vi "Get Pole Orientations.vi"(11 "Pole":bool[](array[boolean])) -> (1 "Pole Swap Options Negative":T1, 3 "Pole Swap Options Positive":T1)   [LabVIEW 2018]
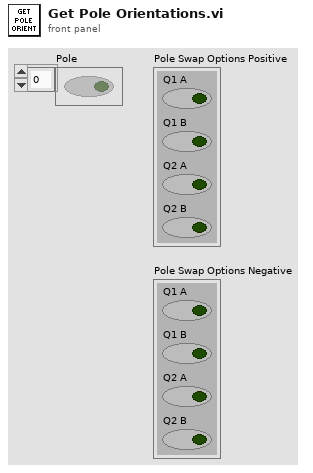
[diagram p1: front panel]
types:
  T1 = cluster{"Q1 A":bool, "Q1 B":bool, "Q2 A":bool, "Q2 B":bool}
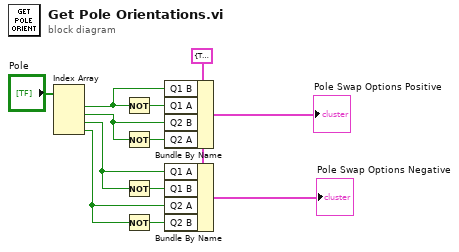
[diagram p0: block diagram]
diagram:
  w12 = T1 {"Q1 A"=TRUE, "Q1 B"=FALSE, "Q2 A"=TRUE, "Q2 B"=FALSE} ("Pole Swap Options Positive")
  n1 = Index Array(array="Pole") -> (element #1=w3:bool, element #2=w5:bool, element #3=w7:bool, element #4=w8:bool)  [unwired: 4 in]
  n2 = Not(x=w3) -> (.not. x?=w4:bool)
  n3 = Not(x=w5) -> (.not. x?=w6:bool)
  n4 = Not(x=w7) -> (.not. x?=w9:bool)
  n5 = Not(x=w8) -> (.not. x?=w10:bool)
  n6 = Bundle By Name(cluster=w12, "Q1 B"=w3, "Q1 A"=w4, "Q2 B"=w5, "Q2 A"=w6) -> (→"Pole Swap Options Positive":T1)
  n7 = Bundle By Name(cluster=w12, "Q1 A"=w7, "Q1 B"=w9, "Q2 A"=w8, "Q2 B"=w10) -> (→"Pole Swap Options Negative":T1)
